vi "Specify Panel Blank.vi"(8 "error in (no error)":errorcluster, 9 "Initial Blank Count (0)":i32, 10 "Blank VI":refnum<class "2DPanelBlank.lvclass">, 11 "2DArrayManager in":refnum<class "2DArrayManager.lvclass">) -> (0 "error out":errorcluster, 3 "2DArrayManager out":refnum<class "2DArrayManager.lvclass">)   [LabVIEW 2020, in "OOPanel.lvlib" / "2DArrayManager.lvclass"]
uses:
  2DArrayManager.lvclass
  2DPanelBlank/2DPanelBlank.lvclass
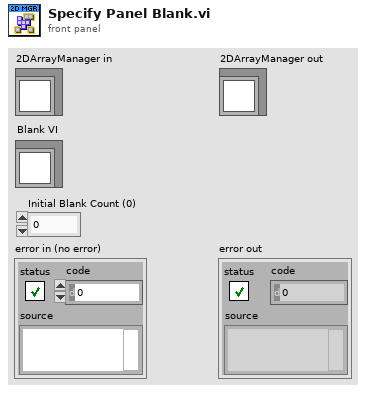
[diagram p1: front panel]
types:
  T1 = typedef "OOPanel.lvlib/2DArrayManager.lvclass/Options.ctl" = cluster{"Running":bool, "Borders":bool, "Background":u32, "V Scroll":bool, "H Scroll":bool, "Blank":refnum<class "2DPanelBlank.lvclass">, "Initial Blank Count":i32}
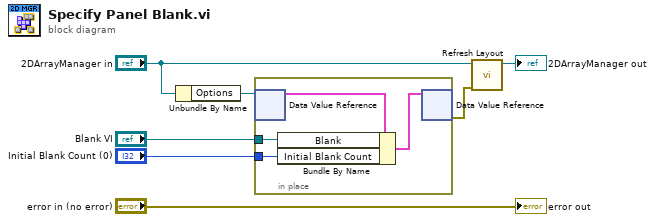
[diagram p0: block diagram]
diagram:
  n1 = Unbundle By Name("2DArrayManager in") -> ("Options"=w6:refnum<data-value>)
  n2 = in-place {
    in-place-border: "Blank VI" -> [w9]
    in-place-border: "Initial Blank Count (0)" -> [w8]
    n3 = in-place-dvr #1(w6) -> (w11:T1)  [unwired: 1 out]
    n4 = Bundle By Name(cluster=w11, "Blank"=w9, "Initial Blank Count"=w8) -> (w10:T1)
    n5 = in-place-dvr #1(w10) -> (w2:errorcluster)  [unwired: 1 out]
  }
  n6 = call "Refresh Layout.vi"("error in (no error)"=w2, "2DArrayManager in"="2DArrayManager in") -> ("2DArrayManager out"=→"2DArrayManager out":refnum<class "2DArrayManager.lvclass">)  [unwired: 8 in, 1 out]
  "error out" <- "error in (no error)"
